vi "send to pc.vi"() -> ()   [LabVIEW 2011, in "talk.lvrbt"]
uses:
  talk.lvrbt
  <vilib>/NXT/Block Support/NXT_MessageMailbox.ctl
  <vilib>/NXT/Dual Mode Library/BT/BlueTooth_Write_Num_toComputer.vi
  <vilib>/NXT/Dual Mode Library/Display/drawNumber.vi
panel:
  in  "stop":bool
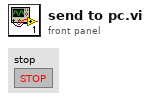
[diagram p1: front panel]
types:
  T1 = typedef "NXT_MessageMailbox.ctl" = u8
  T2 = typedef "LVHSConnector.ctl" = cluster{"Hardware":string, "Flattened String":string}
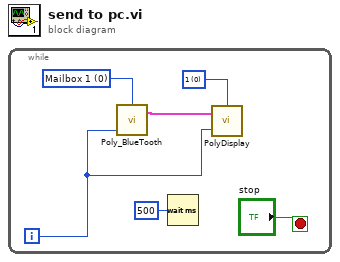
[diagram p0: block diagram]
diagram:
  n1 = while {
    i -> [w3]
    stop <- "stop" stop-if-true
    w4 = i16 0 items=["1", "2", "3", "4", "5", "6", "7", "8"] ("Line")
    w6 = T1 0 items=["Mailbox 1", "Mailbox 2", "Mailbox 3", "Mailbox 4", "Mailbox 5", "Mailbox 6", "Mailbox 7", "Mailbox 8", "Mailbox 9", "Mailbox 10"] ("Mailbox")
    n2 = call-poly <vilib>:"Poly_BlueTooth.vi"("Message in"=w3, "Mailbox"=w6) -> ("NXT"=w5:T2)  [unwired: 2 in]
    n3 = Wait (ms)(milliseconds to wait=u32 500) -> ()  [unwired: 1 out]
    n4 = call-poly <vilib>:"PolyDisplay.vi"("number"=w3, "NXT"=w5, "Line"=w4) -> ()  [unwired: 1 in, 1 out]
  }
